vi "Write Configuration Name.vi"(8 "error in":errorcluster, 10 "Configuration Name":string, 11 "PL_System Configuration in":refnum<class "PL_System Configuration.lvclass">) -> (0 "error out":errorcluster, 3 "PL_System Configuration out":refnum<class "PL_System Configuration.lvclass">)   [LabVIEW 2013, in "PL_System Configuration.lvclass"]
uses:
  PL_System Configuration.lvclass
  <vilib>/NI/Configuration Framework/serializable configuration/NISE_CEF_serializable configuration.lvclass
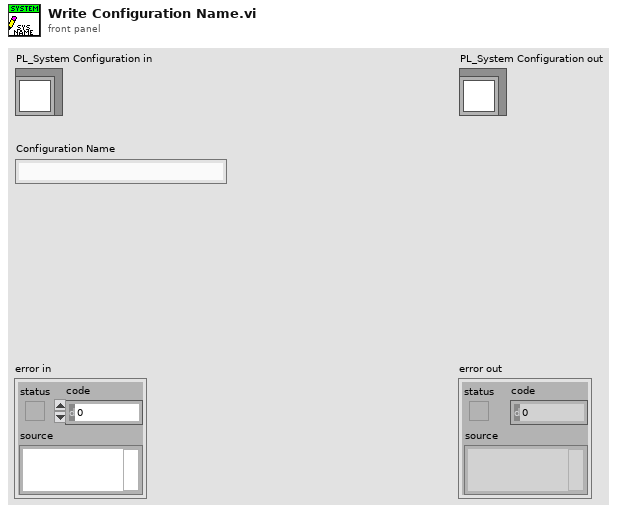
[diagram p1: front panel]
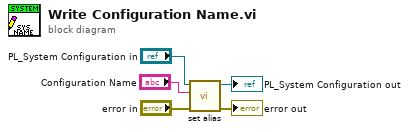
[diagram p0: block diagram]
diagram:
  n1 = call <vilib>:"set alias.vi"("error in"="error in", "alias"="Configuration Name", "configuration in"="PL_System Configuration in") -> ("error out"=→"error out":errorcluster, "configuration out"=→"PL_System Configuration out":refnum<class "PL_System Configuration.lvclass">)  [unwired: 7 in]
